vi "Pack welcome byte.vi"(3 "Serliaser":T1=1 items=["JSON"=1, "MessagePack"=2], 4 "Length (octets)":u8 format="%x") -> (2 "Bytes":u8[](array[numeric]))   [LabVIEW 2020, in "wamplv.lvlib" / "RawSocket Handler.lvclass"]
uses:
  RawSocket Handler.lvclass
  Serilisation Types.ctl
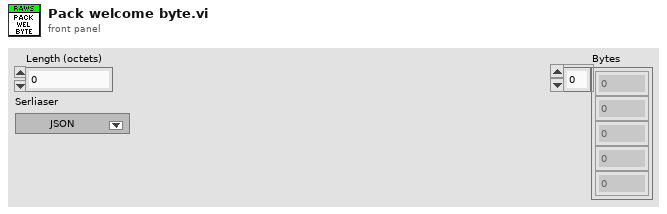
[diagram p1: front panel]
types:
  T1 = typedef "wamplv.lvlib/RawSocket Handler.lvclass/Serilisation Types.ctl" = u8
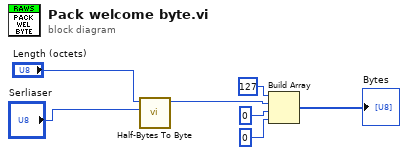
[diagram p0: block diagram]
diagram:
  n1 = call "Half-Bytes To Byte.vi"("Lower Half-byte"="Serliaser", "Upper Half-Byte"="Length (octets)") -> ("Byte"=w2:u8)  [unwired: 7 in]
  n2 = Build Array(u8 127, w2, u8 0 ("element"), u8 0 ("element")) -> (→"Bytes":u8[])
